vi "MT_channels.vi"(8 "error in":errorcluster) -> (0 "error out":errorcluster, 3 "task out":refnum<k21>)   [LabVIEW 2019]
uses:
  <vilib>/DAQmx/create/channels.llb/DAQmx Create Channel (AI-Voltage-Basic).vi
  <vilib>/DAQmx/configure/timing.llb/DAQmx Timing (Sample Clock).vi
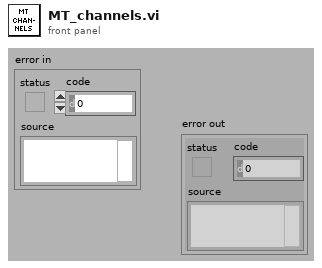
[diagram p1: front panel]
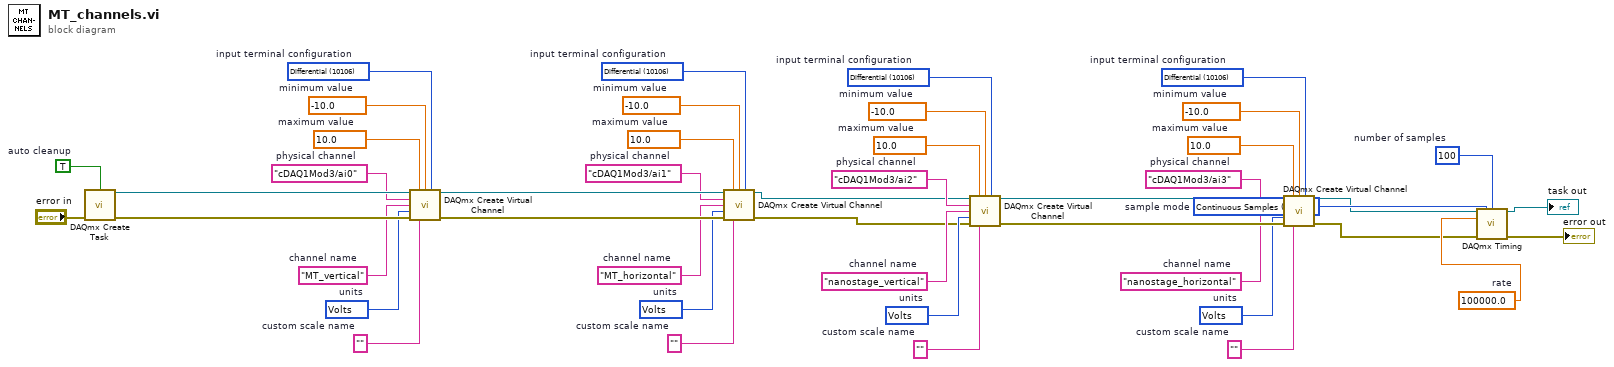
[diagram p0: block diagram]
diagram:
  w5 = 10106 items=["default"=-1, "RSE"=10083, "NRSE"=10078, "Differential"=10106, "Pseudodifferential"=12529]  # input terminal configuration
  w6 = 10348 items=["Volts"=10348, "From Custom Scale"=10065]  # units
  w7 = "nanostage_horizontal"  # channel name
  w8 = ""  # custom scale name
  w9 = -10.0  # minimum value
  w10 = 10.0  # maximum value
  w11 = "cDAQ1Mod3/ai3"  # physical channel
  w13 = 10106 items=["default"=-1, "RSE"=10083, "NRSE"=10078, "Differential"=10106, "Pseudodifferential"=12529]  # input terminal configuration
  w14 = 10348 items=["Volts"=10348, "From Custom Scale"=10065]  # units
  w15 = "nanostage_vertical"  # channel name
  w17 = ""  # custom scale name
  w18 = -10.0  # minimum value
  w19 = 10.0  # maximum value
  w20 = "cDAQ1Mod3/ai2"  # physical channel
  w21 = 10123 items=["Finite Samples"=10178, "Continuous Samples"=10123, "Hardware Timed Single Point"=12522]  # sample mode
  w22 = 100  # number of samples
  w23 = 100000.0  # rate
  w26 = 10106 items=["default"=-1, "RSE"=10083, "NRSE"=10078, "Differential"=10106, "Pseudodifferential"=12529]  # input terminal configuration
  w27 = 10348 items=["Volts"=10348, "From Custom Scale"=10065]  # units
  w28 = "MT_horizontal"  # channel name
  w29 = ""  # custom scale name
  w30 = -10.0  # minimum value
  w31 = 10.0  # maximum value
  w32 = "cDAQ1Mod3/ai1"  # physical channel
  w34 = 10106 items=["default"=-1, "RSE"=10083, "NRSE"=10078, "Differential"=10106, "Pseudodifferential"=12529]  # input terminal configuration
  w35 = 10348 items=["Volts"=10348, "From Custom Scale"=10065]  # units
  w36 = "MT_vertical"  # channel name
  w38 = ""  # custom scale name
  w39 = -10.0  # minimum value
  w40 = 10.0  # maximum value
  w41 = "cDAQ1Mod3/ai0"  # physical channel
  w43 = TRUE  # auto cleanup
  n1 = call <vilib>:"DAQmx Create Task.vi"("auto cleanup"=w43, "error in"="error in") -> ("task out"=w42:refnum<k21>, "error out"=w44:errorcluster)  [unwired: 12 in]
  n2 = call-poly <vilib>:"DAQmx Create Virtual Channel.vi"("task in"=w42, "maximum value"=w40, "minimum value"=w39, "input terminal configuration"=w34, "physical channels"=w41, "name to assign"=w36, "units"=w35, "error in"=w44, "custom scale name"=w38) -> ("task out"=w33:refnum<k21>, "error out"=w37:errorcluster)  [unwired: 5 in]
  n3 = call-poly <vilib>:"DAQmx Create Virtual Channel.vi"("task in"=w33, "maximum value"=w31, "minimum value"=w30, "input terminal configuration"=w26, "physical channels"=w32, "name to assign"=w28, "units"=w27, "error in"=w37, "custom scale name"=w29) -> ("task out"=w2:refnum<k21>, "error out"=w1:errorcluster)  [unwired: 5 in]
  n4 = call-poly <vilib>:"DAQmx Create Virtual Channel.vi"("task in"=w2, "maximum value"=w19, "minimum value"=w18, "input terminal configuration"=w13, "physical channels"=w20, "name to assign"=w15, "units"=w14, "error in"=w1, "custom scale name"=w17) -> ("task out"=w12:refnum<k21>, "error out"=w16:errorcluster)  [unwired: 5 in]
  n5 = call-poly <vilib>:"DAQmx Create Virtual Channel.vi"("task in"=w12, "maximum value"=w10, "minimum value"=w9, "input terminal configuration"=w5, "physical channels"=w11, "name to assign"=w7, "units"=w6, "error in"=w16, "custom scale name"=w8) -> ("task out"=w4:refnum<k21>, "error out"=w3:errorcluster)  [unwired: 5 in]
  n6 = call-poly <vilib>:"DAQmx Timing.vi"("task/channels in"=w4, "sample mode"=w21, "samples per channel"=w22, "rate"=w23, "error in"=w3) -> ("task out"=→"task out":refnum<k21>, "error out"=→"error out":errorcluster)  [unwired: 9 in]
